vi "ColorMatch_MainFunction.vi"(8 "error in (no error)":errorcluster, 10 "ColorMatchParameter":T2={"Color Sensitivity"=0, "Learn Saturation Threshold"=80, "Minimum Match Score"=800.0, "Match Saturation Threshold"=80, "ROI Descriptor"={"Global Rectangle"=[], "Contours"=[]}, "TemplatePath"="", "ColorSpectrum"=[]} {"Color Sensitivity" items=["Low", "Medium", "High"]; "ROI Descriptor"."Contours"."Type" items=["No Selection", "Point", "Line", "Rectangle", "Oval", "Polygon", "Freehand Region", "Annulus", "Unused2", "Unused3", "Broken Line", "Freehand Line", "Rotated Rectangle"]}, 11 "Vision_Image In":T1) -> (0 "error out":errorcluster, 2 "Match Score":i32[](array[numeric]), 3 "Match Flag":bool[](array[boolean]))   [LabVIEW 2019]
uses:
  Controls/ColorMatch/Analysis_ColorMatch_Parameter.ctl
  <vilib>/vision/Image Controls.llb/IMAQ Image.ctl
  <vilib>/vision/NI_Vision_Development_Module.lvlib
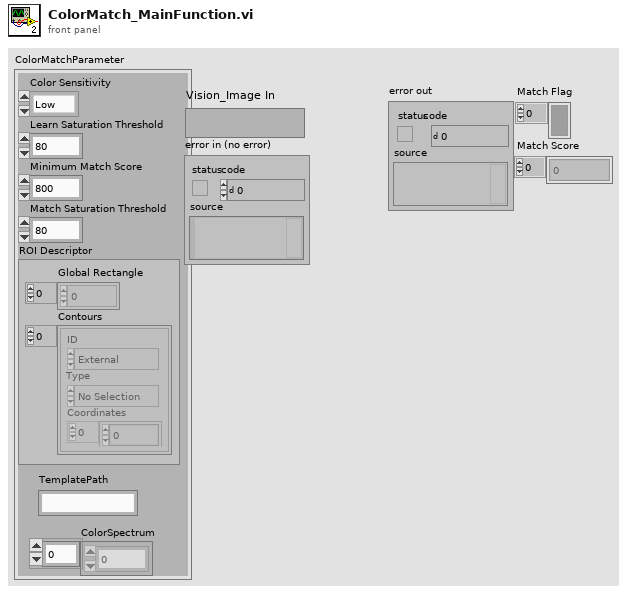
[diagram p1: front panel]
types:
  T1 = typedef "IMAQ Image.ctl" = refnum<image>
  T2 = typedef "Analysis_ColorMatch_Parameter.ctl" = cluster{"Color Sensitivity":u32, "Learn Saturation Threshold":i32, "Minimum Match Score":dbl, "Match Saturation Threshold":i32, "ROI Descriptor":T3, "TemplatePath":string, "ColorSpectrum":dbl[]}
  T3 = typedef "ROI Descriptor" = cluster{"Global Rectangle":i32[], "Contours":cluster{"ID":enum32{"External", "Internal"}, "Type":u32, "Coordinates":i32[]}[]}
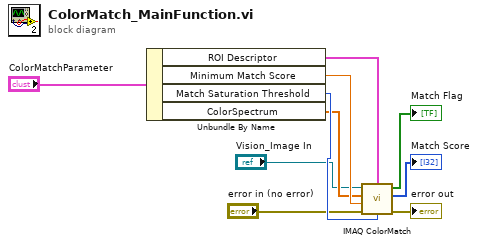
[diagram p0: block diagram]
diagram:
  n1 = Unbundle By Name("ColorMatchParameter") -> ("ROI Descriptor"=w9:T3, "Minimum Match Score"=w8:dbl, "Match Saturation Threshold"=w7:i32, "ColorSpectrum"=w6:dbl[])
  n2 = call "IMAQ ColorMatch"("ROI Descriptor"=w9, "Image"="Vision_Image In", "Color Spectrum"=w6, "Match Saturation Threshold"=w7, "Minimum Match Score"=w8, "error in (no error)"="error in (no error)") -> ("Match Flag"=→"Match Flag":bool[], "Match Score"=→"Match Score":i32[], "error out"=→"error out":errorcluster)  [unwired: 1 out]
